vi "zc internal encoding from data.vi"(8 "error in (no error)":errorcluster, 10 "data":cluster{}, 11 "this_":cluster{}) -> (0 "error out":errorcluster, 3 "this_ out":cluster{})   [LabVIEW 2021, in "zenohc.lvlib"]
doc: "void zc_internal_encoding_from_data(struct z_owned_encoding_t *this_,\n struct zc_internal_encoding_data_t data);"
uses:
  zenohc.lvlib
  zenohc.dll
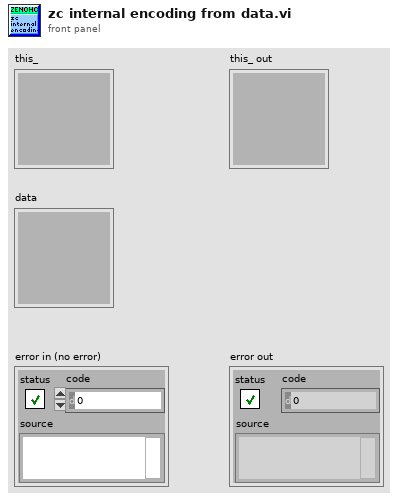
[diagram p1: front panel]
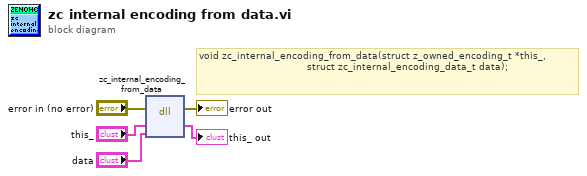
[diagram p0: block diagram]
diagram:
  # "void zc_internal_encoding_from_data(struct z_owned_encoding_t *this_,\n                                    struct zc_internal_encoding_data_t data);"
  n1 = dll-call lib="D:/dev/zenoh_labview/zenohc/zenohc.*" fn="zc_internal_encoding_from_data"(error in="error in (no error)", "this_"="this_", "data"="data") -> (error out=→"error out":errorcluster, "this_"=→"this_ out":cluster{})  [unwired: 4 in, 1 out]
